vi "Set Zero Point.vi"(8 "error in (no error)":errorcluster, 9 "firmware revision":string(combo), 10 "zero point":T1={"capacitance (0)"=0.0, "loss (0)"=0.0, "frequency (1000)"=1000.0}, 11 "VISA resource name":refnum<visa-resource-name>) -> (0 "error out":errorcluster, 2 "bridge error":T2, 3 "VISA resource name out":refnum<visa-resource-name>)   [LabVIEW 2024, in "Andeen-Hagerling 2700A.lvlib"]
doc: "Provides a manual way to enter capacitance and loss Zero\ncompensation values."
uses:
  Andeen-Hagerling 2700A.lvlib
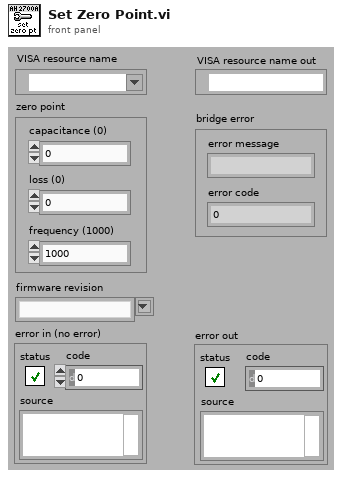
[diagram p1: front panel]
types:
  T1 = cluster{"capacitance (0)":dbl, "loss (0)":dbl, "frequency (1000)":dbl}
  T2 = cluster{"error message":string, "error code":i32}
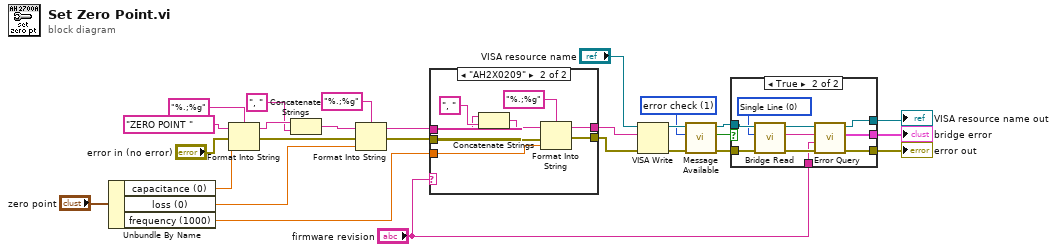
[diagram p0: block diagram]
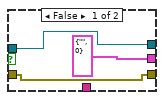
[diagram p2: hidden frame]
diagram:
  w1 = u16 1 items=["none", "error check", "multiline read", "infinite"] ("delay")
  n1 = Unbundle By Name("zero point") -> ("capacitance (0)"=w4:dbl, "loss (0)"=w3:dbl, "frequency (1000)"=w2:dbl)
  n2 = Format Into String(format string="%.;%g", initial string="ZERO POINT " ("command"), error in="error in (no error)", w4) -> (resulting string=w24:string, error out=w25:errorcluster)
  n3 = Concatenate Strings(w24, ", " ("command")) -> (w20:string)
  n4 = Format Into String(format string="%.;%g", initial string=w20, error in=w25, w3) -> (resulting string=w18:string, error out=w17:errorcluster)
  n5 = case shown="\"AH2X0209\"" "firmware revision" {
    tunnel: w18 -> [w29 w34]
    tunnel: w17 -> [w28 w33]
    tunnel: [w28 w32] -> w16
    tunnel: [w29 w31] -> w15
    tunnel: w2 -> [_ w30]
    frame "AH2X0208", Default {
    }
    frame "AH2X0209" {
      n6 = Concatenate Strings(w34, ", " ("command")) -> (w36:string)
      n7 = Format Into String(format string="%.;%g", initial string=w36, error in=w33, w30) -> (resulting string=w31:string, error out=w32:errorcluster)
    }
  }
  n8 = VISA Write(VISA resource name="VISA resource name", write buffer=w15, error in (no error)=w16) -> (VISA resource name out=w11:refnum<visa-resource-name>, error out=w10:errorcluster)  [unwired: 1 out]
  n9 = call "Message Available.vi"("error in (no error)"=w10, "delay"=w1, "VISA resource name"=w11) -> ("error out"=w12:errorcluster, "message available"=w14:bool, "VISA resource name out"=w13:refnum<visa-resource-name>)  [unwired: 6 in]
  n10 = case shown="True" w14 {
    tunnel: w13 -> [w39 w47]
    tunnel: w12 -> [w40 w46]
    tunnel: "firmware revision" -> [_ w45]
    tunnel: [w40 w44] -> w9
    tunnel: [w39 w43] -> w8
    tunnel: [T2 {"error message"="", "error code"=0} ("bridge error") w42] -> w6
    frame False {
    }
    frame True {
      w41 = u16 0 items=["Single Line", "Multi-Line"] ("Multiline")
      n11 = call "Bridge Read.vi"("error in (no error)"=w46, "multiline"=w41, "VISA resource name"=w47) -> ("error out"=w49:errorcluster, "read buffer"=w50:string, "VISA resource name out"=w48:refnum<visa-resource-name>)  [unwired: 6 in]
      n12 = call "Error Query.vi"("error in (no error)"=w49, "firmware revision"=w45, "measurement line"=w50, "VISA resource name"=w48) -> ("error out"=w44:errorcluster, "bridge error"=w42:T2, "VISA resource name out"=w43:refnum<visa-resource-name>)  [unwired: 5 in]
    }
  }
  "VISA resource name out" <- w8
  "error out" <- w9
  "bridge error" <- w6
